vi "信号持续时间参数配置.vi"(11 "标题":string) -> ()   [LabVIEW 2016, in "环境动力监测库.lvlib"]
panel:
  in  "信号持续时间":u32=60 format="%.0fS"
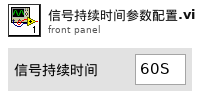
[diagram p1: front panel]
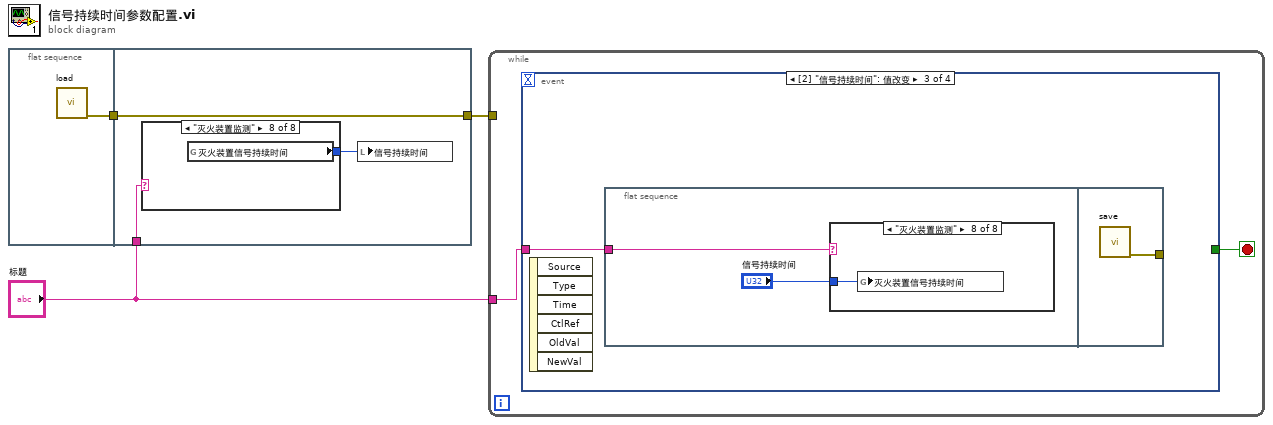
[diagram p0: block diagram]
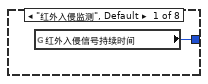
[diagram p2: hidden frame]
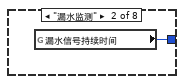
[diagram p3: hidden frame]
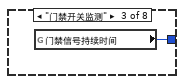
[diagram p4: hidden frame]
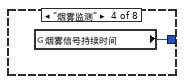
[diagram p5: hidden frame]
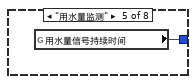
[diagram p6: hidden frame]
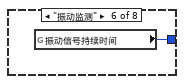
[diagram p7: hidden frame]
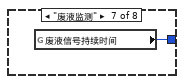
[diagram p8: hidden frame]
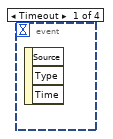
[diagram p9: hidden frame]
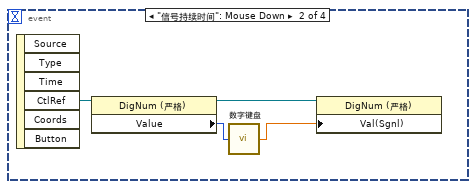
[diagram p10: hidden frame]
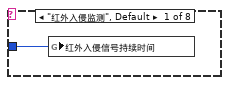
[diagram p11: hidden frame]
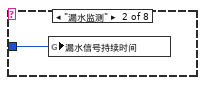
[diagram p12: hidden frame]
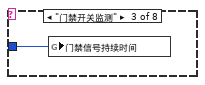
[diagram p13: hidden frame]
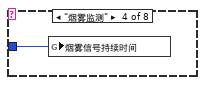
[diagram p14: hidden frame]
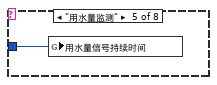
[diagram p15: hidden frame]
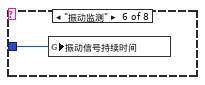
[diagram p16: hidden frame]
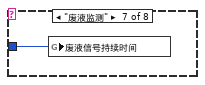
[diagram p17: hidden frame]
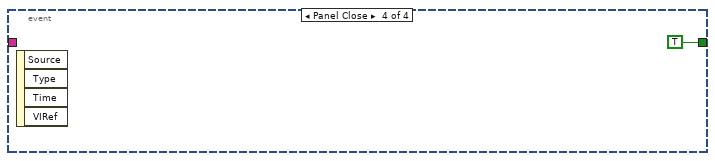
[diagram p18: hidden frame]
diagram:
  n1 = flat-sequence {
    tunnel: [w4] -> w3
    tunnel: [w7] -> w2
    tunnel: w3 -> [w7]
    tunnel: "标题" -> [w5]
    frame #0 {
      n2 = call "load.vi"() -> ("error out"=w4:errorcluster)  [unwired: 11 in]
    }
    frame #1 {
      n3 = case shown="\"灭火装置监测\"" w5 {
        tunnel: [w8 w9 w10 w11 w12 w13 w14 w15] -> w6
        frame "红外入侵监测", Default {
          n4 = global read "断电保存全局变量.vi" "红外入侵信号持续时间"() -> (w8:u32)
        }
        frame "漏水监测" {
          n5 = global read "断电保存全局变量.vi" "漏水信号持续时间"() -> (w9:u32)
        }
        frame "门禁开关监测" {
          n6 = global read "断电保存全局变量.vi" "门禁信号持续时间"() -> (w10:u32)
        }
        frame "烟雾监测" {
          n7 = global read "断电保存全局变量.vi" "烟雾信号持续时间"() -> (w11:u32)
        }
        frame "用水量监测" {
          n8 = global read "断电保存全局变量.vi" "用水量信号持续时间"() -> (w12:u32)
        }
        frame "振动监测" {
          n9 = global read "断电保存全局变量.vi" "振动信号持续时间"() -> (w13:u32)
        }
        frame "废液监测" {
          n10 = global read "断电保存全局变量.vi" "废液信号持续时间"() -> (w14:u32)
        }
        frame "灭火装置监测" {
          n11 = global read "断电保存全局变量.vi" "灭火装置信号持续时间"() -> (w15:u32)
        }
      }
      n12 = local write "信号持续时间"(w6) -> ()
    }
  }
  n13 = while {
    tunnel: w2 -> [_]
    tunnel: "标题" -> [w16]
    stop <- w17 stop-if-true
    n14 = event shown="[2] \"信号持续时间\": 值改变" {
      selector: _ -> [_ _ _ _]
      dyn-events: _ -> [_ _ _ _]
      timeout: _ -> [_ _ _ _]
      tunnel: [_ _ _ TRUE] -> w17
      tunnel: w16 -> [_ _ w22 _]
      event Timeout {
        n15 = event-data() -> ()  [unwired: 1 in, 3 out]
      }
      event "信号持续时间": Mouse Down {
        n16 = event-data() -> ("CtlRef"=w18:refnum<vi>)  [unwired: 1 in, 5 out]
        n17 = property class="DigNum (严格)"(reference=w18) -> (reference out=w20:refnum<vi>, "Value"=w21:u32)  [unwired: 1 in, 1 out]
        n18 = call "数字键盘.vi"("OldNumber"=w21) -> ("NewNumber"=w19:sgl)
        n19 = property class="DigNum (严格)"(reference=w20, "Val(Sgnl)"=w19) -> ()  [unwired: 1 in, 2 out]
      }
      event "信号持续时间": Value Change {
        n20 = event-data() -> ()  [unwired: 1 in, 6 out]
        n21 = flat-sequence {
          tunnel: w22 -> [w24]
          tunnel: [w33] -> _
          frame #0 {
            n22 = case shown="\"灭火装置监测\"" w24 {
              tunnel: "信号持续时间" -> [w25 w26 w27 w28 w29 w30 w31 w32]
              frame "红外入侵监测", Default {
                n23 = global write "断电保存全局变量.vi" "红外入侵信号持续时间"(w25) -> ()
              }
              frame "漏水监测" {
                n24 = global write "断电保存全局变量.vi" "漏水信号持续时间"(w26) -> ()
              }
              frame "门禁开关监测" {
                n25 = global write "断电保存全局变量.vi" "门禁信号持续时间"(w27) -> ()
              }
              frame "烟雾监测" {
                n26 = global write "断电保存全局变量.vi" "烟雾信号持续时间"(w28) -> ()
              }
              frame "用水量监测" {
                n27 = global write "断电保存全局变量.vi" "用水量信号持续时间"(w29) -> ()
              }
              frame "振动监测" {
                n28 = global write "断电保存全局变量.vi" "振动信号持续时间"(w30) -> ()
              }
              frame "废液监测" {
                n29 = global write "断电保存全局变量.vi" "废液信号持续时间"(w31) -> ()
              }
              frame "灭火装置监测" {
                n30 = global write "断电保存全局变量.vi" "灭火装置信号持续时间"(w32) -> ()
              }
            }
          }
          frame #1 {
            n31 = call "save.vi"() -> ("error out"=w33:errorcluster)  [unwired: 11 in]
          }
        }
      }
      event Panel Close {
        n32 = event-data() -> ()  [unwired: 1 in, 4 out]
      }
    }
  }
